vi "New Container.vi"(0 "Session Handle in":T2, 11 "error in (no error)":errorcluster) -> (4 "Session Handle out":T2, 6 "New Value Container":T1, 15 "error out":errorcluster)   [LabVIEW 2019, in "HTS.lvlib" / "Engine.lvclass"]
uses:
  Engine.lvclass
  VariableContainer/VariableContainer.lvclass
  Typedefs/Session Handle.ctl
  VariableContainer/Typedefs/Session Handle.ctl
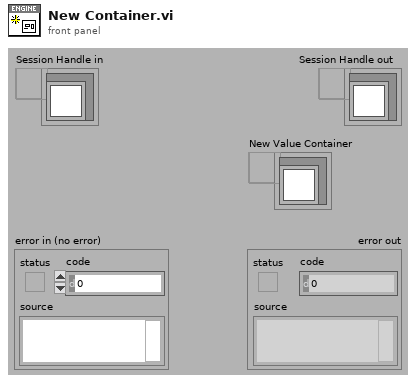
[diagram p1: front panel]
types:
  T1 = typedef "HTS.lvlib/VariableContainer.lvclass/Session Handle.ctl" = refnum<data-value>
  T2 = typedef "HTS.lvlib/Engine.lvclass/Session Handle.ctl" = refnum<data-value>
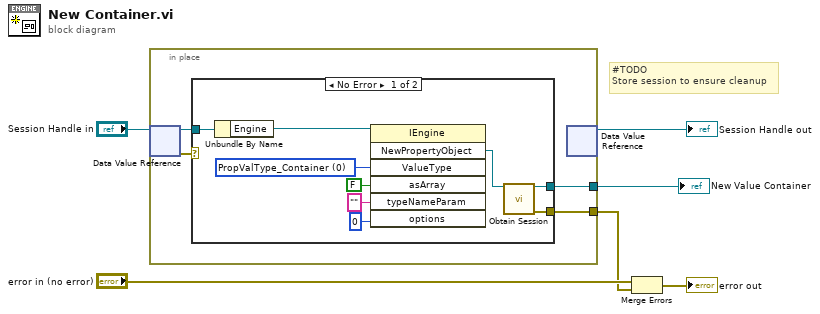
[diagram p0: block diagram]
diagram:
  # "#TODO\nStore session to ensure cleanup"
  n1 = in-place {
    in-place-border: [w8] -> w4
    in-place-border: [w7] -> w2
    n2 = in-place-dvr #1("Session Handle in") -> (w10:refnum<class "Engine.lvclass">, w9:errorcluster)
    n3 = case shown="No Error" w9 {
      selector: w9 -> [_ w20]
      tunnel: w10 -> [w19 _]
      tunnel: [w15 _] -> w8
      tunnel: [w14 w20] -> w7
      frame No Error {
        w17 = 0 items=["PropValType_Container", "PropValType_String", "PropValType_Boolean", "PropValType_Number", "PropValType_NamedType", "PropValType_Reference", "PropValType_Array", "PropValType_Enum"] ("ValueType")
        n4 = Unbundle By Name(w19) -> ("Engine"=w18:refnum<k7>)
        n5 = invoke class="IEngine" method="NewPropertyObject"(reference=w18, "ValueType"=w17, "asArray"=FALSE, "typeNameParam"="", "options"=0) -> ("NewPropertyObject"=w16:refnum<k7>)  [unwired: 2 in, 6 out]
        n6 = call "Obtain Session.vi"("PropertyObject"=w16) -> ("Session Handle"=w15:T1, "error out"=w14:errorcluster)  [unwired: 13 in]
      }
      frame Error {
      }
    }
    n7 = in-place-dvr #1() -> (→"Session Handle out":T2)  [unwired: 1 in, 1 out]
  }
  "New Value Container" <- w4
  n8 = Merge Errors("error in (no error)", w2) -> (→"error out":errorcluster)
